vi "Get references (SubVI).vi"(0 "TestSocketName in":string) -> (4 "MISO CO.Pulse.Term":tag, 6 "MISO":tag, 8 "CLK":tag, 10 "MOSI":tag, 15 "CS":tag)   [LabVIEW 2023, in "SPI.lvlib"]
uses:
  SPI.lvlib
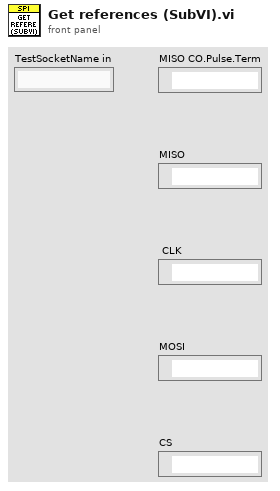
[diagram p1: front panel]
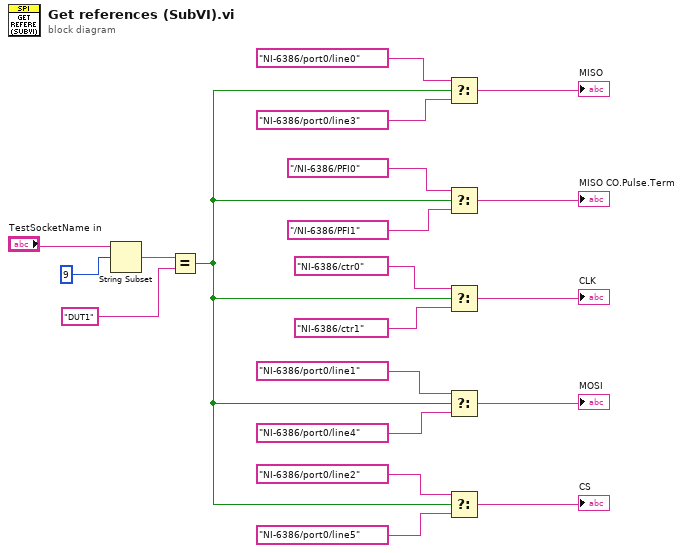
[diagram p0: block diagram]
diagram:
  n1 = String Subset(string="TestSocketName in", offset (0)=9) -> (substring=w17:string)  [unwired: 1 in]
  n2 = Equal?(x=w17, y="DUT1") -> (x = y?=w1:bool)
  n3 = Select(t=tag "NI-6386/port0/line0" ("lines"), s=w1, f=tag "NI-6386/port0/line3" ("lines")) -> (s? t:f=→"MISO":tag)
  n4 = Select(t=tag "/NI-6386/PFI0" ("CO.Pulse.Term"), s=w1, f=tag "/NI-6386/PFI1" ("CO.Pulse.Term")) -> (s? t:f=→"MISO CO.Pulse.Term":tag)
  n5 = Select(t=tag "NI-6386/ctr0" ("lines"), s=w1, f=tag "NI-6386/ctr1" ("lines")) -> (s? t:f=→"CLK":tag)
  n6 = Select(t=tag "NI-6386/port0/line1" ("lines"), s=w1, f=tag "NI-6386/port0/line4" ("lines")) -> (s? t:f=→"MOSI":tag)
  n7 = Select(t=tag "NI-6386/port0/line2" ("lines"), s=w1, f=tag "NI-6386/port0/line5" ("lines")) -> (s? t:f=→"CS":tag)
